vi "test counter outputs crds.vi"() -> ()   [LabVIEW 2012]
uses:
  <vilib>/DAQmx/configure/timing.llb/DAQmx Timing (Implicit).vi
  <resource>/objmgr/daqmx.rc
panel:
  out "error out":errorcluster
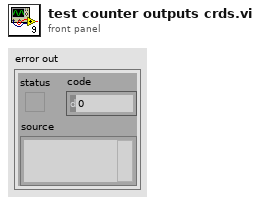
[diagram p1: front panel]
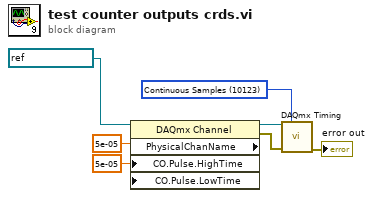
[diagram p0: block diagram]
diagram:
  w7 = 10123 items=["Finite Samples"=10178, "Continuous Samples"=10123, "Hardware Timed Single Point"=12522] ("sample mode")
  n1 = property class="DAQmx Channel" props=["PhysicalChanName", "CO.Pulse.HighTime", "CO.Pulse.LowTime"](reference=refnum<k21> "CRD Diode" ("Diode CO"), "CO.Pulse.HighTime"=5e-05 ("CO.Pulse.DutyCyc"), "CO.Pulse.LowTime"=5e-05 ("CO.Pulse.Freq")) -> (reference out=w6:refnum<k21>, error out=w5:errorcluster)  [unwired: 1 in, 1 out]
  n2 = call-poly <vilib>:"DAQmx Timing.vi"("task/channels in"=w6, "sample mode"=w7, "error in"=w5) -> ("error out"=→"error out":errorcluster)  [unwired: 11 in, 1 out]
